vi "sc_initSerial.vi"(8 "error in (no error)":errorcluster, 11 "VISA resource name":refnum<visa-resource-name>) -> (0 "error out":errorcluster, 2 "initialization error":bool, 3 "VISA resource name out":refnum<visa-resource-name>)   [LabVIEW 2015]
uses:
  <vilib>/Instr/_visa.llb/VISA Configure Serial Port (Instr).vi
  <vilib>/Instr/_visa.llb/VISA Open Access Mode.ctl
  controls/scientifica_commands.ctl
panel:
  out "Response":string
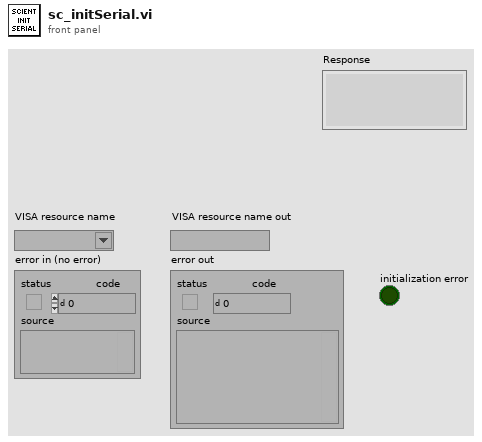
[diagram p1: front panel]
types:
  T1 = typedef "scientifica_commands.ctl" = enum16{"ANGLE", "INSET", "FIRST", "ZERO", "Pz", "P", "absz", "ACC", "TOP", "STOP", "rel", "relz", "abs", "IN", "vj", "APROACH", "OBJS", "OBJU", "OUT", "OBJ", "OBJL", "SET", "OBJD", "STEP", "SETSTEP", "S", "UUX", "UUY", "UUZ"}
  T2 = typedef "VISA Open Access Mode.ctl" = u32
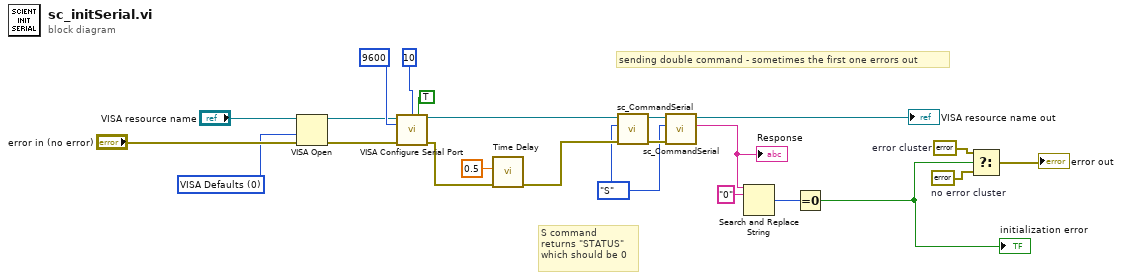
[diagram p0: block diagram]
diagram:
  w6 = errorcluster {"status"=TRUE, "code"=0, "source"="Scientifica actuator not properly initialized!"}  # error cluster
  w7 = errorcluster {"status"=FALSE, "code"=0, "source"=""}  # no error cluster
  w2 = scientifica_commands."S" ("Scientifica commands")
  w18 = T2 0 items=["VISA Defaults"=0, "Exclusive Lock"=1, "Load Configured Settings"=4] ("Access Mode")
  # "S command\nreturns \"STATUS\"\nwhich should be 0"
  # "sending double command - sometimes the first one errors out"
  n1 = VISA Open(access mode=w18, error in (no error)="error in (no error)", VISA resource name="VISA resource name") -> (VISA resource name=w22:refnum<visa-resource-name>, error out=w21:errorcluster)  [unwired: 2 in]
  n2 = call-poly "VISA Configure Serial Port"("VISA resource name"=w22, "termination char\n(0xA = '\\n' = LF)"=u8 10 ("termination char\n(0xA = '\\n' = LF)"), "Enable Termination\nChar (T)"=TRUE ("Enable Termination\nChar (T)"), "baud rate (9600)"=u32 9600, "error in (no error)"=w21) -> ("VISA resource name out"=w1:refnum<visa-resource-name>, "error out"=w13:errorcluster)  [unwired: 9 in]
  n3 = call "Time Delay"("error in (no error)"=w13, "Delay Time (s)"=0.5) -> ("error out"=w5:errorcluster)  [unwired: 9 in]
  n4 = call "sc_CommandSerial.vi"("error in (no error)"=w5, "Scientifica commands"=w2, "VISA handle"=w1) -> ("error out"=w4:errorcluster, "Dup. VISA handle"=w3:refnum<visa-resource-name>)  [unwired: 5 in, 2 out]
  n5 = call "sc_CommandSerial.vi"("error in (no error)"=w4, "Scientifica commands"=w2, "VISA handle"=w3) -> ("Response"=w12:string, "Dup. VISA handle"=→"VISA resource name out":refnum<visa-resource-name>)  [unwired: 5 in, 2 out]
  "Response" <- w12
  n6 = Search and Replace String(input string=w12, search string="0") -> (number of replacements=w10:i32)  [unwired: 6 in, 3 out]
  n7 = Equal To 0?(x=w10) -> (x = 0?=w9:bool)
  "initialization error" <- w9
  n8 = Select(t=w6, s=w9, f=w7) -> (s? t:f=→"error out":errorcluster)
